vi "AutoPowerMesa.vi"() -> ()   [LabVIEW 2015]
panel:
  out "EOff":string
  out "EOn":string
  out "IOff":string
  out "IOn":string
  in  "VISA resource name":refnum<visa-resource-name>="COM11"
  in  "EnOff":bool
  in  "EnOn":bool
  in  "IgnOff":bool
  in  "IgnOn":bool
  in  "stop":bool
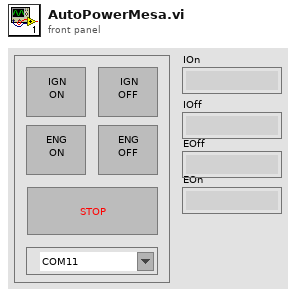
[diagram p1: front panel]
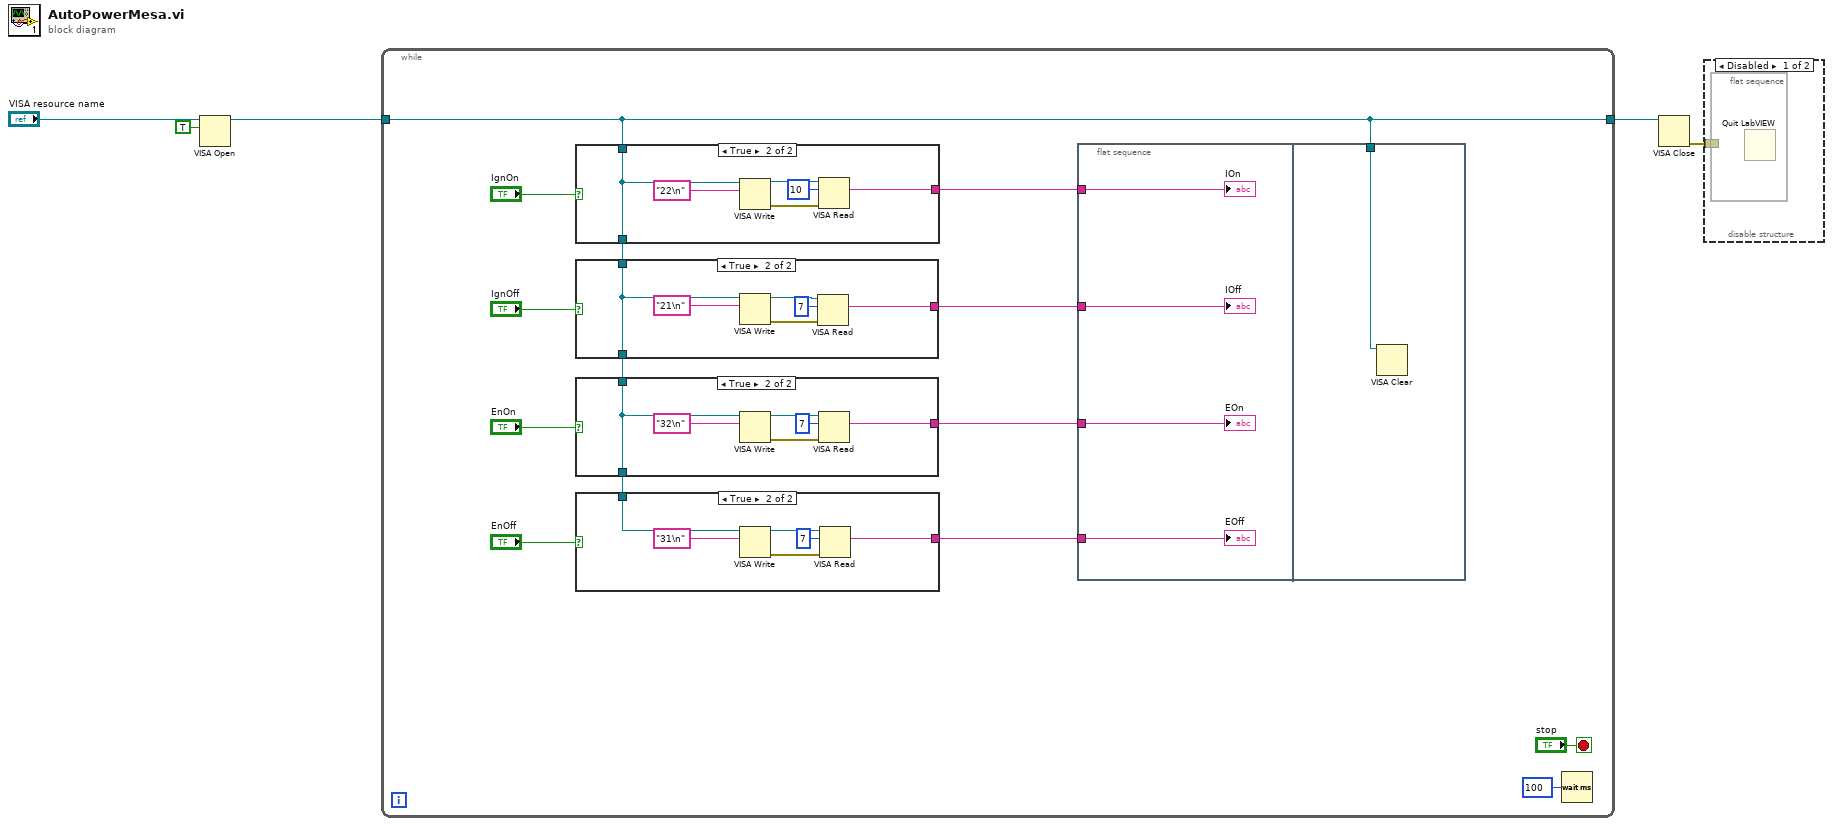
[diagram p0: block diagram]
diagram:
  n1 = VISA Open(duplicate session (F)=TRUE, VISA resource name="VISA resource name") -> (VISA resource name=w3:refnum<visa-resource-name>)  [unwired: 3 in, 1 out]
  n2 = while {
    tunnel: w3 -> [w6]
    tunnel: [w6] -> w5
    stop <- "stop" stop-if-true
    n3 = case shown="True" "IgnOn" {
      tunnel: w6 -> [w45 w50]
      tunnel: [w45 w50] -> w17
      tunnel: [_ w47] -> w10
      frame False {
      }
      frame True {
        n4 = VISA Write(VISA resource name=w50, write buffer="22\n") -> (VISA resource name out=w49:refnum<visa-resource-name>, error out=w48:errorcluster)  [unwired: 1 in, 1 out]
        n5 = VISA Read(VISA resource name=w49, byte count=u32 10, error in (no error)=w48) -> (read buffer=w47:string)  [unwired: 3 out]
      }
    }
    n6 = case shown="True" "IgnOff" {
      tunnel: w17 -> [w38 w43]
      tunnel: [w38 w43] -> w14
      tunnel: [_ w39] -> w9
      frame False {
      }
      frame True {
        n7 = VISA Write(VISA resource name=w43, write buffer="21\n") -> (VISA resource name out=w41:refnum<visa-resource-name>, error out=w40:errorcluster)  [unwired: 1 in, 1 out]
        n8 = VISA Read(VISA resource name=w41, byte count=u32 7, error in (no error)=w40) -> (read buffer=w39:string)  [unwired: 3 out]
      }
    }
    n9 = case shown="True" "EnOn" {
      tunnel: w14 -> [w31 w36]
      tunnel: [w31 w36] -> w15
      tunnel: [_ w32] -> w8
      frame False {
      }
      frame True {
        n10 = VISA Write(VISA resource name=w36, write buffer="32\n") -> (VISA resource name out=w34:refnum<visa-resource-name>, error out=w33:errorcluster)  [unwired: 1 in, 1 out]
        n11 = VISA Read(VISA resource name=w34, byte count=u32 7, error in (no error)=w33) -> (read buffer=w32:string)  [unwired: 3 out]
      }
    }
    n12 = case shown="True" "EnOff" {
      tunnel: w15 -> [_ w29]
      tunnel: [_ w25] -> w7
      frame False {
      }
      frame True {
        n13 = VISA Write(VISA resource name=w29, write buffer="31\n") -> (VISA resource name out=w27:refnum<visa-resource-name>, error out=w26:errorcluster)  [unwired: 1 in, 1 out]
        n14 = VISA Read(VISA resource name=w27, byte count=u32 7, error in (no error)=w26) -> (read buffer=w25:string)  [unwired: 3 out]
      }
    }
    n15 = flat-sequence {
      tunnel: w10 -> [w23]
      tunnel: w9 -> [w22]
      tunnel: w8 -> [w21]
      tunnel: w7 -> [w20]
      tunnel: w6 -> [w24]
      frame #0 {
        "IOn" <- w23
        "IOff" <- w22
        "EOn" <- w21
        "EOff" <- w20
      }
      frame #1 {
        n16 = VISA Clear(VISA resource name=w24) -> ()  [unwired: 1 in, 2 out]
      }
    }
    n17 = Wait (ms)(milliseconds to wait=u32 100) -> ()  [unwired: 1 out]
  }
  n18 = VISA Close(VISA resource name=w5) -> (error out=w4:errorcluster)  [unwired: 1 in]
  n19 = disable-structure shown="Disabled" {
    disable-tunnel: w4 -> [w52 _]
    frame Disabled {
      n20 = flat-sequence {
        tunnel: w52 -> [_]
        frame #0 {
          n21 = Quit LabVIEW() -> ()  [unwired: 1 in]
        }
      }
    }
    frame Enabled {
    }
  }
